vi "Get Default QD Object Shortcuts File.vi"() -> (2 "file exists":bool, 3 "default shortcuts text file":path)   [LabVIEW 2016]
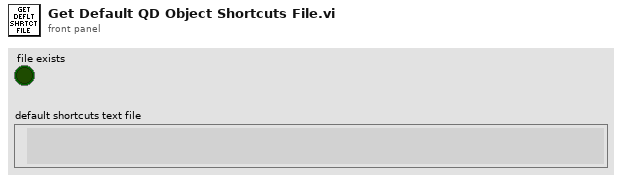
[diagram p1: front panel]
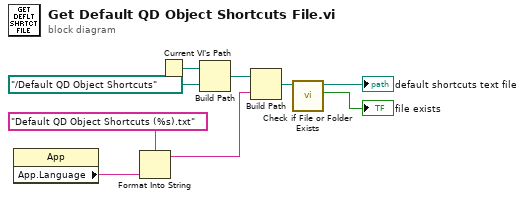
[diagram p0: block diagram]
diagram:
  n1 = property class="App"() -> ("App.Language"=w1:string)  [unwired: 2 in, 2 out]
  n2 = Format Into String(format string="Default QD Object Shortcuts (%s).txt", w1) -> (resulting string=w3:string)  [unwired: 2 in, 1 out]
  n3 = Current VI's Path() -> (path=w7:path)
  n4 = Build Path(base path=w7, name or relative path=path "../Default QD Object Shortcuts") -> (appended path=w8:path)
  n5 = Build Path(base path=w8, name or relative path=w3) -> (appended path=w4:path)
  n6 = call <vilib>:"Check if File or Folder Exists.vi"("path"=w4) -> ("file or folder exists?"=→"file exists":bool, "dup path"=→"default shortcuts text file":path)  [unwired: 8 in, 1 out]
